vi "FRCts20_WebMethods_Division_GET.vi"(7 "httpRequestID":u32, 10 "division":string, 11 "competition":string) -> ()   [LabVIEW 2013, in "FRCts20_WebMethods.lvlib"]
doc: "<B>GET</B> on the specified <B>division</B> resource\n\nhttp://<server address>:<port>/FRCts/competition/<B>competition</B>/division/<B>division</B>"
uses:
  FRCts20_WebMethods.lvlib
  <vilib>/wsapi/NI_WebServices.lvlib
  Backend/source/VI Source/FRCts20_Backend_API/FRCts20_Backend_API_SW.ctl
  Backend/source/VI Source/FRCts20_Backend_API/FRCts20_Backend_API.lvlib
  Backend/source/VI Source/FRCts20_Backend_API/FRCts20_Backend_API_Division.ctl
  Backend/source/VI Source/FRCts20_Backend_API/FRCts20_Backend_API_Command_Division.ctl
  Backend/source/VI Source/FRCts20_Backend_API/FRCts20_Backend_API_Status.ctl
  Backend/source/VI Source/FRCts20_Backend_API/FRCts20_Backend_API_Event.vi
panel:
  in  "query":string
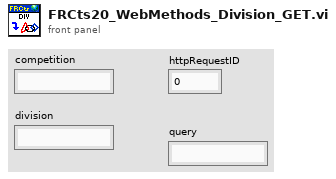
[diagram p1: front panel]
types:
  T1 = typedef "FRCts20_Backend_API.lvlib/FRCts20_Backend_API_Command_Division.ctl" = string
  T2 = typedef "FRCts20_Backend_API.lvlib/FRCts20_Backend_API_Division.ctl" = cluster{"Location":string, "Team":u32[], "APIReturn":string, "RootCmd":enum16{"Issues", "Software", "All"}, "SWType":T3, "Status":T4, "Competition":string}
  T3 = typedef "FRCts20_Backend_API.lvlib/FRCts20_Backend_API_SW.ctl" = string
  T4 = typedef "FRCts20_Backend_API.lvlib/FRCts20_Backend_API_Status.ctl" = enum16{"Open", "In Work", "Closed"}
  T5 = typedef "FRCts20_Backend_API.lvlib/FRCts20_Backend_API_Event.ctl" = cluster{"Event Index":u32, "Name":string, "Start Time":timestamp, "End Time":timestamp, "Teams":cluster{"Team Index":u32, "Team Number":u32, "Requests":cluster{"Request Number":u32, "Description":string}[], "Has Open Issue":bool}[], "SWType":T3, "APIReturn":string}
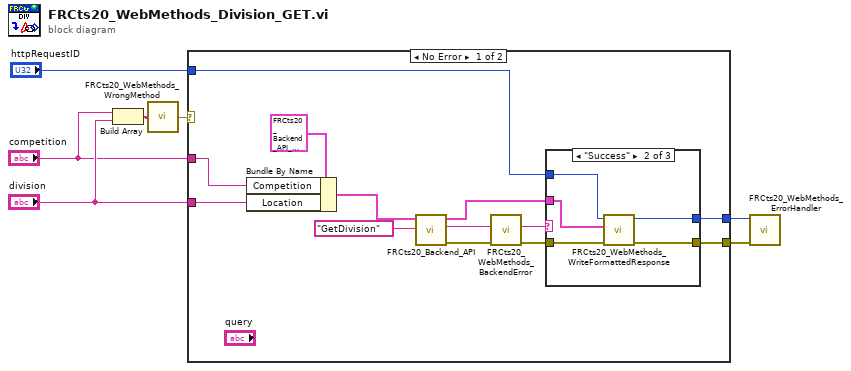
[diagram p0: block diagram]
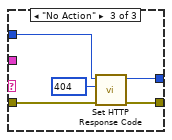
[diagram p3: hidden frame]
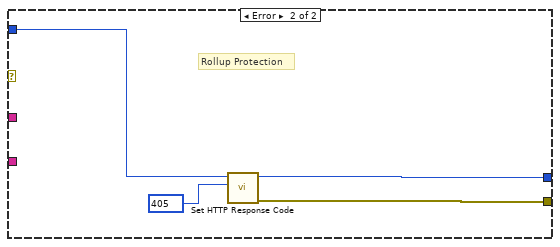
[diagram p4: hidden frame]
diagram:
  n1 = Build Array("competition", "division") -> (w6:string[])
  n2 = call "FRCts20_WebMethods_WrongMethod.vi"(4:w6) -> (1:w7)  [unwired: 3 in, 1 out]
  n3 = case shown="No Error" w7 {
    tunnel: "httpRequestID" -> [w11 w36]
    tunnel: [w9 w34] -> w3
    tunnel: [w8 w33] -> w4
    tunnel: "division" -> [w19 _]
    tunnel: "competition" -> [w18 _]
    frame No Error {
      n4 = Bundle By Name(cluster=T2 {"Location"="", "Team"=[], "APIReturn"="", "RootCmd"=enum."Issues", "SWType"="", "Status"=enum."Open", "Competition"=""} ("Division"), "Competition"=w18, "Location"=w19) -> (w17:T2)
      n5 = call-poly "FRCts20_Backend_API.vi"("Command"=T1 "GetDivision", "Event In"=w17) -> ("error out"=w15:errorcluster, "Status"=w14:string, "Event Out"=w10:T5)  [unwired: 7 in]
      n6 = call "FRCts20_WebMethods_BackendError.vi"("error in (no error)"=w15, "Status"=w14) -> ("error out"=w12:errorcluster, "Status out"=w13:string)  [unwired: 8 in]
      n7 = case shown="\"Success\"" w13 {
        tunnel: w12 -> [w21 w27 w29]
        tunnel: w11 -> [w22 w26 w30]
        tunnel: w10 -> [_ w25 _]
        tunnel: [w22 w24 w31] -> w9
        tunnel: [w21 w23 w32] -> w8
        frame "Backend Error", Default {
        }
        frame "Success" {
          n8 = call "FRCts20_WebMethods_WriteFormattedResponse.vi"("error in (no error)"=w27, "Response Cluster"=w25, "httpRequestID"=w26) -> ("error out"=w23:errorcluster, "httpRequestID out"=w24:u32)  [unwired: 7 in]
        }
        frame "No Action" {
          w28 = 404 items=["100"=100, "101"=101, "200"=200, "201"=201, "202"=202, "203"=203, "204"=204, "205"=205, "206"=206, "300"=300, "301"=301, "302"=302, "303"=303, "304"=304, "305"=305, "306"=306, "307"=307, "400"=400, "401"=401, "402"=402, "403"=403, "404"=404, "405"=405, "406"=406, "407"=407, "408"=408, "409"=409, "410"=410, "411"=411, "412"=412, "413"=413, "414"=414, "415"=415, "416"=416, "417"=417, "500"=500, "501"=501, "502"=502, "503"=503, "504"=504, "505"=505] ("response code (200)")
          n9 = call <vilib>:"Set HTTP Response Code.vi"("error in (no error)"=w29, "response code (200)"=w28, "httpRequestID"=w30) -> ("error out"=w32:errorcluster, "httpRequestID out"=w31:u32)  [unwired: 7 in]
        }
      }
    }
    frame Error {
      w35 = 405 items=["100"=100, "101"=101, "200"=200, "201"=201, "202"=202, "203"=203, "204"=204, "205"=205, "206"=206, "300"=300, "301"=301, "302"=302, "303"=303, "304"=304, "305"=305, "306"=306, "307"=307, "400"=400, "401"=401, "402"=402, "403"=403, "404"=404, "405"=405, "406"=406, "407"=407, "408"=408, "409"=409, "410"=410, "411"=411, "412"=412, "413"=413, "414"=414, "415"=415, "416"=416, "417"=417, "500"=500, "501"=501, "502"=502, "503"=503, "504"=504, "505"=505] ("response code (200)")
      # "Rollup Protection"
      n10 = call <vilib>:"Set HTTP Response Code.vi"("response code (200)"=w35, "httpRequestID"=w36) -> ("error out"=w33:errorcluster, "httpRequestID out"=w34:u32)  [unwired: 8 in]
    }
  }
  n11 = call "FRCts20_WebMethods_ErrorHandler.vi"("error in"=w4, "httpRequestID"=w3) -> ()  [unwired: 9 in, 1 out]
